vi "Generate-S-Box.vi"() -> ()   [LabVIEW 2017]
panel:
  out "S-Box":u8[](array[numeric]) format="%.0x"
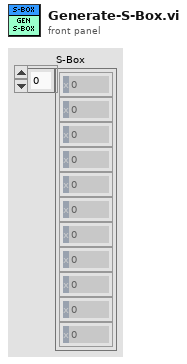
[diagram p1: front panel]
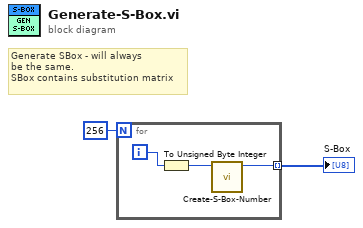
[diagram p0: block diagram]
diagram:
  # "Generate SBox - will always \nbe the same.\nSBox contains substitution matrix"
  n1 = for {
    N: 256 -> [_]
    tunnel: [w4] -> w1 mode=indexing
    i -> [w5]
    n2 = To Unsigned Byte Integer(number=w5) -> (unsigned 8bit integer=w3:u8)
    n3 = call "Create-S-Box-Number.vi"("Index"=w3) -> ("S-Box"=w4:u8)  [unwired: 10 in]
  }
  "S-Box" <- w1
